vi "toNextDay.vi"(11 "Cron in":T1) -> (3 "Cron out":T1)   [LabVIEW 2013, in "openCron.lvlib" / "Cron.lvclass"]
uses:
  Cron.lvclass
  CronTime -- cluster.ctl
  <vilib>/LabVIEW Open Source Project/Epoch Date & Time/GregorianCal_Month -- enum.ctl
  <vilib>/LabVIEW Open Source Project/Epoch Date & Time/GregorianCal_MonthLengths.vi
  <vilib>/LabVIEW Open Source Project/Epoch Date & Time/isLeapYear (integer).vi
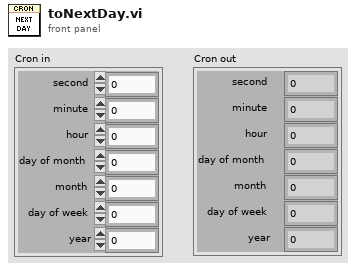
[diagram p1: front panel]
types:
  T1 = typedef "openCron.lvlib/Cron.lvclass/CronTime -- cluster.ctl" = cluster{"second":i32, "minute":i32, "hour":i32, "day of month":i32, "month":i32, "day of week":i32, "year":i32}
  T2 = typedef "GregorianCal_Month -- enum.ctl" = enum16{"January", "February", "March", "April", "May", "June", "July", "August", "September", "October", "November", "December"}
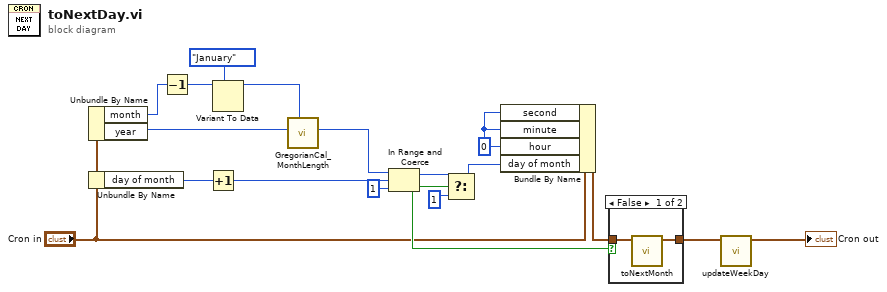
[diagram p0: block diagram]
diagram:
  w13 = 0 ("hour")
  n1 = Unbundle By Name("Cron in") -> ("month"=w7:i32, "year"=w9:i32)
  n2 = Unbundle By Name("Cron in") -> ("day of month"=w18:i32)
  n3 = Decrement(x=w7) -> (x-1=w3:i32)
  n4 = Increment(x=w18) -> (x+1=w17:i32)
  n5 = Variant To Data(type=GregorianCal_Month_--_enum."January" ("Month"), Variant=w3) -> (data=w5:T2)  [unwired: 1 in, 1 out]
  n6 = call <vilib>:"GregorianCal_MonthLength.vi"("Month"=w5, "Year (0: this year)"=w9) -> ("Nb Days"=w4:i32)  [unwired: 9 in]
  n7 = In Range and Coerce(upper limit=w4, x=w17, lower limit=1) -> (coerced(x)=w15:i32, In Range?=w11:bool)
  n8 = Select(t=w15, s=w11, f=1 ("month")) -> (s? t:f=w10:i32)
  n9 = Bundle By Name(cluster="Cron in", "second"=w13, "minute"=w13, "hour"=w13, "day of month"=w10) -> (w12:T1)
  n10 = case shown="False" w11 {
    tunnel: w12 -> [w20 w21]
    tunnel: [w19 w21] -> w1
    frame False {
      n11 = call "toNextMonth.vi"("Cron in"=w20) -> ("Cron out"=w19:T1)  [unwired: 10 in]
    }
    frame True {
    }
  }
  n12 = call "updateWeekDay.vi"("Cron in"=w1) -> ("Cron Time"=→"Cron out":T1)  [unwired: 10 in]
